vi "CC Focus Generate Channel List.vi"(8 "error in (no error)":errorcluster) -> (0 "error out":errorcluster, 1 "Channel Names":string[](array[string])=["Telescope RA", "Telescope DEC", "Telescope Moving?", "Telescope Status"], 3 "Channel List":refnum<class "HK Item.lvclass">[](array[class]))   [LabVIEW 2024]
uses:
  hk-channel-class/hk-channel-class/HK Item/HK Item.lvclass
  hk-channel-class/hk-channel-class/HK Item/HK Channel Units and Setup.ctl
  hk-channel-class/hk-channel-class/HK Item/HK Channel enum Data Type.ctl
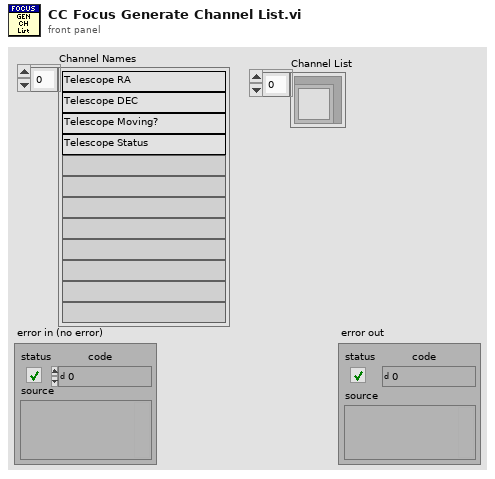
[diagram p1: front panel]
types:
  T1 = typedef "HK Item.lvclass/HK Channel Units and Setup.ctl" = cluster{"Unit Type":string, "Units":string, "Configuration":string, "Digits":i32, "Data Type":T2, "Exponential?":bool, "Source":string}
  T2 = typedef "HK Item.lvclass/HK Channel enum Data Type.ctl" = enum16{"Floating Point", "Integer", "Enum", "String", "Waveform", "File"}
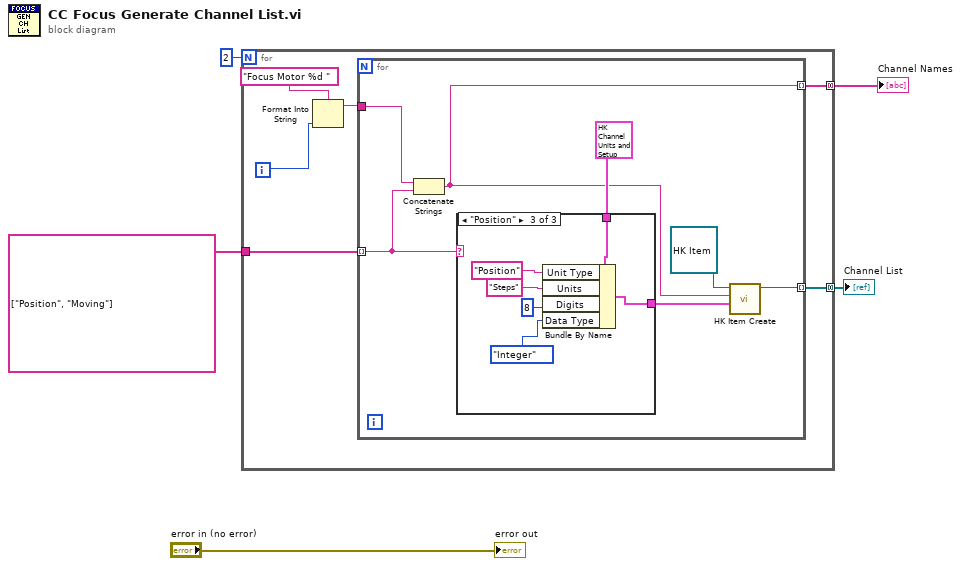
[diagram p0: block diagram]
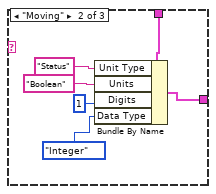
[diagram p3: hidden frame]
diagram:
  n1 = for {
    N: 2 -> [_]
    tunnel: string[] ["Position", "Moving"] -> [w11]
    tunnel: [w10] -> w3 mode=concatenating
    tunnel: [w9] -> w2 mode=concatenating
    i -> [w6]
    n2 = Format Into String(format string="Focus Motor %d ", w6) -> (resulting string=w8:string)  [unwired: 2 in, 1 out]
    n3 = for {
      tunnel: w11 -> [w13] mode=indexing
      tunnel: [w16] -> w10 mode=indexing
      tunnel: w8 -> [w14]
      tunnel: [w12] -> w9 mode=indexing
      n4 = Concatenate Strings(w14, w13) -> (w12:string)
      n5 = case shown="\"Position\"" w13 {
        tunnel: T1 {"Unit Type"="", "Units"="", "Configuration"="", "Digits"=3, "Data Type"=enum."Floating Point", "Exponential?"=FALSE, "Source"=""} ("Channel Setup") -> [w19 w25 w31]
        tunnel: [w19 w20 w26] -> w18
        frame "False", Default {
        }
        frame "Moving" {
          n6 = Bundle By Name(cluster=w25, "Unit Type"="Status", "Units"="Boolean", "Digits"=1, "Data Type"=HK_Channel_enum_Data_Type."Integer") -> (w20:T1)
        }
        frame "Position" {
          n7 = Bundle By Name(cluster=w31, "Unit Type"="Position", "Units"="Steps", "Digits"=8, "Data Type"=HK_Channel_enum_Data_Type."Integer") -> (w26:T1)
        }
      }
      n8 = call-dynamic "HK Item Create.vi"("Channel Setup"=w18, "Name"=w12, "HK Item in"=refnum<class "HK Item.lvclass"> refnum) -> ("HK Item out"=w16:refnum<class "HK Item.lvclass">)  [unwired: 7 in, 1 out]
    }
  }
  "Channel List" <- w3
  "Channel Names" <- w2
  "error out" <- "error in (no error)"
